vi "Check Label.vi"(11 "Label":string) -> (3 "Boolean":bool)   [LabVIEW 2017]
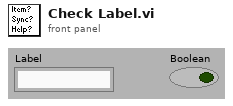
[diagram p1: front panel]
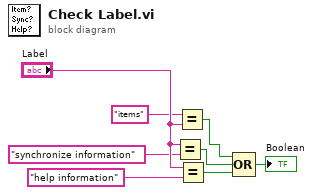
[diagram p0: block diagram]
diagram:
  n1 = Equal?(x="Label", y="synchronize information") -> (x = y?=w5:bool)
  n2 = Equal?(x="items" ("y"), y="Label") -> (x = y?=w6:bool)
  n3 = Equal?(x="Label", y="help information") -> (x = y?=w1:bool)
  n4 = Compound Arithmetic op=OR(w6, w5, w1) -> (→"Boolean":bool)
